vi "test Error Wrapping - Sets Error For Inner Error.vi"(8 "error in (no error)":errorcluster, 11 "TestCase in":refnum<class "Error Tests.lvclass">) -> (0 "error out":errorcluster, 3 "TestCase out":refnum<class "Error Tests.lvclass">)   [LabVIEW 2020, in "Error Tests.lvclass"]
uses:
  Error Tests.lvclass
  <vilib>/Utility/file.llb/Application Directory.vi
  <vilib>/Utility/libraryn.llb/Check if File or Folder Exists.vi
  <vilib>/addons/_JKI Toolkits/VI Tester/TestCase.llb/TestCase.lvclass
  C:/Program Files/National Instruments/LabVIEW 2024/vi.lib/addons/_JKI Toolkits/VI Tester/TestCase.llb/TestCase.lvclass
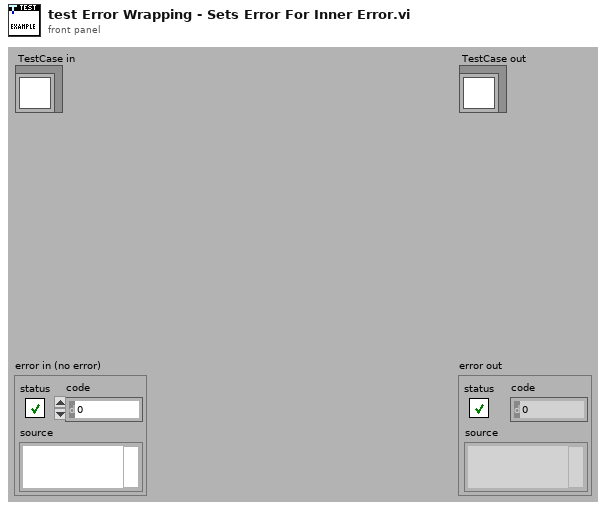
[diagram p1: front panel]
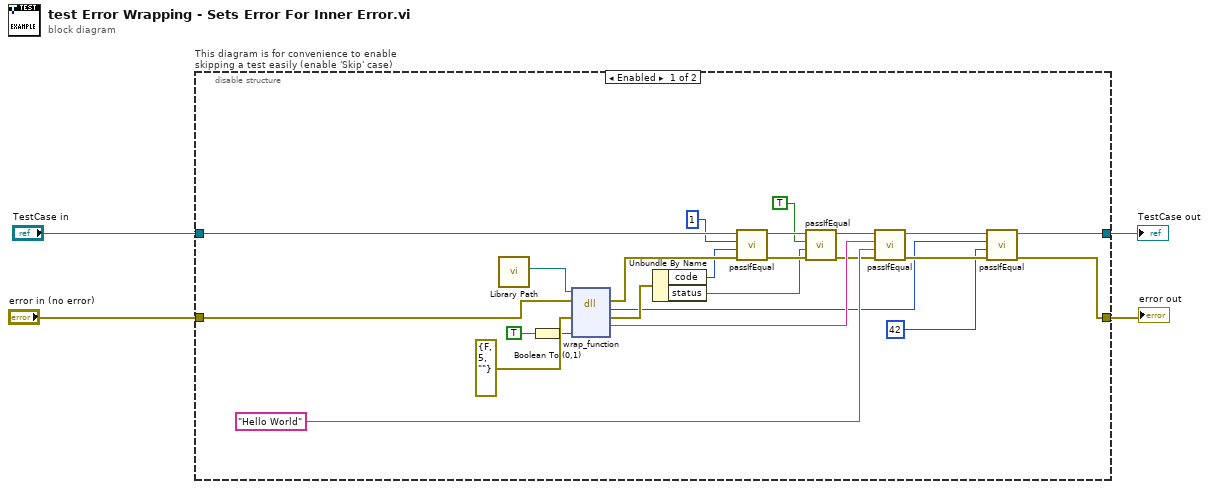
[diagram p0: block diagram]
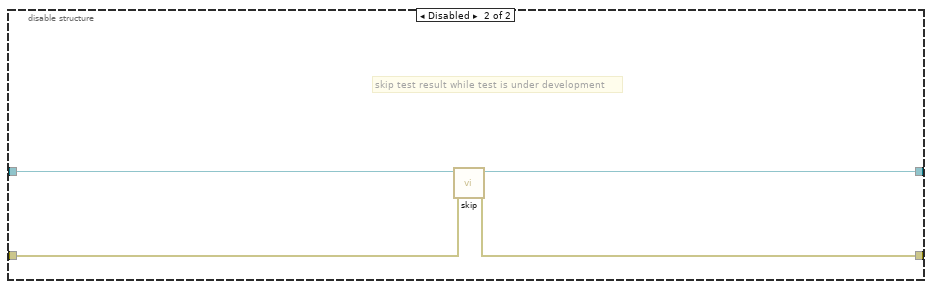
[diagram p2: hidden frame]
diagram:
  n1 = disable-structure "This diagram is for convenience to enable skipping a test easily (enable 'Skip' case)" shown="Enabled" {
    disable-tunnel: "TestCase in" -> [w21 w32]
    disable-tunnel: [w16 w30] -> w1
    disable-tunnel: [w18 w31] -> w3
    disable-tunnel: "error in (no error)" -> [w23 w29]
    frame Enabled {
      n2 = call "Library Path.vi"() -> ("Library Path"=w28:path)  [unwired: 11 in]
      n3 = Boolean To (0,1)(Boolean=TRUE) -> (0, 1=w5:i16)
      n4 = dll-call lib="C:/Users/JamesMcNally/Documents/RustInterop/Rust-LabVIEW-Interop/target/debug/labview_test_library.dll" fn="wrap_function"(path in=w28, error in=w23, "code"=errorcluster {"status"=FALSE, "code"=5, "source"=""} ("error in (no error)"), "inner_error"=w5) -> (error out=w26:errorcluster, "return type"=w15:i32, "code"=w19:errorcluster, "text"=w25:string)  [unwired: 3 in, 1 out]
      n5 = Unbundle By Name(w19) -> ("code"=w12:i32, "status"=w7:bool)
      n6 = call-dynamic "passIfEqual.vi"("error in (no error)"=w26, "y"=w12, "x"=1 ("code"), "TestCase in"=w21) -> ("error out"=w22:errorcluster, "TestCase out"=w9:refnum<class "Error Tests.lvclass">)  [unwired: 6 in]
      n7 = call-dynamic "passIfEqual.vi"("error in (no error)"=w22, "y"=w7, "x"=TRUE ("status"), "TestCase in"=w9) -> ("error out"=w10:errorcluster, "TestCase out"=w8:refnum<class "Error Tests.lvclass">)  [unwired: 6 in]
      n8 = call-dynamic "passIfEqual.vi"("error in (no error)"=w10, "y"="Hello World", "x"=w25, "TestCase in"=w8) -> ("error out"=w27:errorcluster, "TestCase out"=w17:refnum<class "Error Tests.lvclass">)  [unwired: 6 in]
      n9 = call-dynamic "passIfEqual.vi"("error in (no error)"=w27, "y"=42 ("return type"), "x"=w15, "TestCase in"=w17) -> ("error out"=w18:errorcluster, "TestCase out"=w16:refnum<class "Error Tests.lvclass">)  [unwired: 6 in]
    }
    frame Disabled {
      # "skip test result while test is under development"
      n10 = call <vilib>:"skip.vi"("error in (no error)"=w29, "TestCase in"=w32) -> ("error out"=w31:errorcluster, "TestCase out"=w30:refnum<class "Error Tests.lvclass">)  [unwired: 8 in]
    }
  }
  "error out" <- w3
  "TestCase out" <- w1
